vi "Get Pin Map Path.vi"(8 "error in":errorcluster, 10 "Pin Map Relative Path":string, 11 "Sequence Context In":refnum<k7>) -> (0 "error out":errorcluster, 3 "Pin Map Path":string)   [LabVIEW 2020, in "NIDCPowerSourceDCVoltage.lvlib"]
uses:
  NIDCPowerSourceDCVoltage.lvlib
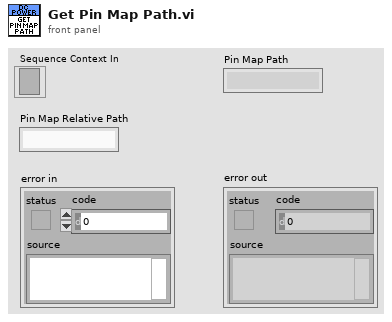
[diagram p1: front panel]
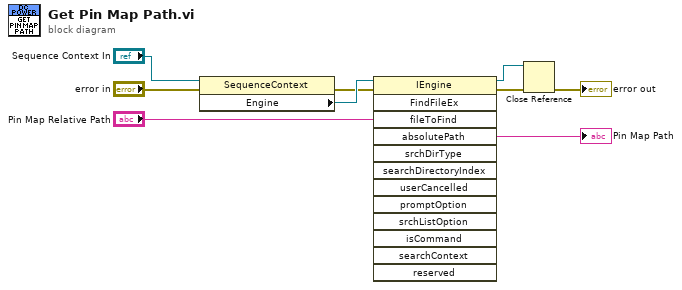
[diagram p0: block diagram]
diagram:
  n1 = property class="SequenceContext"(reference="Sequence Context In", error in="error in") -> (error out=w5:errorcluster, "Engine"=w6:refnum<k7>)  [unwired: 1 out]
  n2 = invoke class="IEngine" method="FindFileEx"(reference=w6, error in=w5, "fileToFind"="Pin Map Relative Path") -> (reference out=w2:refnum<k7>, error out=w1:errorcluster, "absolutePath"=→"Pin Map Path":string)  [unwired: 10 in, 10 out]
  n3 = Close Reference(reference=w2, error in (no error)=w1) -> (error out=→"error out":errorcluster)
